vi "Radau5_Step and Stage Value Calculation.vi"(8 "Y(k)":dbl[](array[numeric]), 9 "Increment Z":dbl[](array[numeric]), 10 "Step size":dbl, 11 "Width":i32) -> (0 "Stage value of Y":dbl[][](array[numeric]), 1 "Stage value of Y'":dbl[][](array[numeric]), 2 "Y(k+1) out":dbl[](array[numeric]), 3 "Y'(k+1) out":dbl[](array[numeric]))   [LabVIEW 2020, in "NI_DAE.lvlib"]
uses:
  <vilib>/gmath/NI_DAE.lvlib
  <vilib>/Analysis/Matrix/Datatypes/RealMatrix.ctl
  <vilib>/Analysis/Matrix/Numeric/Multiply/Multiply - RM,R.vi
  <vilib>/Analysis/Matrix/NI_Matrix.lvlib
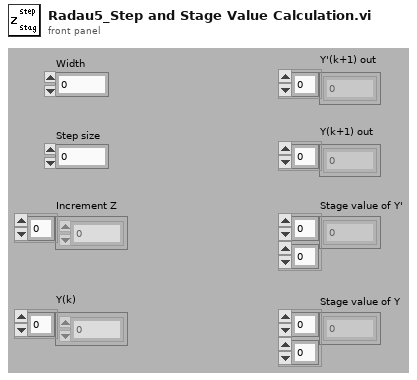
[diagram p1: front panel]
types:
  T1 = typedef "NI_Matrix.lvlib/RealMatrix.ctl" = dbl[][]
  T2 = cluster{"A * c[0]":dbl, "A * c[1]":dbl, "A * c[2]":dbl}
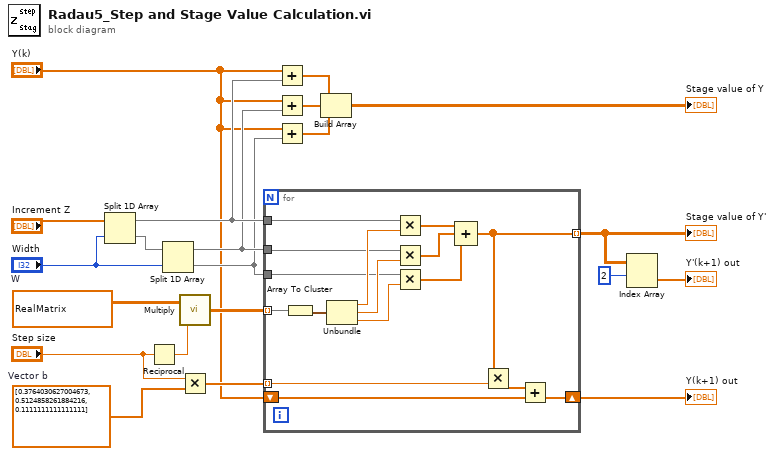
[diagram p0: block diagram]
diagram:
  w8 = dbl[] [0.3764030627004673, 0.5124858261884216, 0.1111111111111111]  # Vector b
  w21 = T1 [[3.2247448713915894, 1.1678400846904053, -0.2531972647421808], [-3.5678400846904057, 0.775255128608411, 1.053197264742181], [5.5319726474218065, -7.53197264742181, 5.0]]  # W
  n1 = Split 1D Array(array="Increment Z", index="Width") -> (first subarray=w15:dbl[], second subarray=w16:dbl[])
  n2 = Reciprocal(x="Step size") -> (1/x=w20:dbl)
  n3 = Split 1D Array(array=w16, index="Width") -> (first subarray=w14:dbl[], second subarray=w13:dbl[])
  n4 = call-poly <vilib>:"Multiply.vi"("Real Scalar c"=w20, "Real Matrix A"=w21) -> ("A * c"=w19:T1)
  n5 = Multiply(x="Step size", y=w8) -> (x*y=w7:dbl[])
  n6 = for {
    tunnel: w19 -> [w37] mode=indexing
    tunnel: w15 -> [w33]
    tunnel: w14 -> [w34]
    tunnel: w13 -> [w31]
    tunnel: [w25] -> w4 mode=indexing
    tunnel: w7 -> [w26] mode=indexing
    shift-right: [w23] -> w5
    shift-left: "Y(k)" -> [w22]
    n7 = Array To Cluster(array=w37) -> (cluster=w36:T2)
    n8 = Unbundle(w36) -> ("A * c[0]"=w35:dbl, "A * c[1]"=w32:dbl, "A * c[2]"=w30:dbl)
    n9 = Multiply(x=w33, y=w35) -> (x*y=w29:dbl[])
    n10 = Multiply(x=w34, y=w32) -> (x*y=w28:dbl[])
    n11 = Multiply(x=w31, y=w30) -> (x*y=w27:dbl[])
    n12 = Compound Arithmetic op=ADD(w29, w28, w27) -> (w25:dbl[])
    n13 = Multiply(x=w25, y=w26) -> (x*y=w24:dbl[])
    n14 = Add(x=w24, y=w22) -> (x+y=w23:dbl[])
  }
  "Stage value of Y'" <- w4
  "Y(k+1) out" <- w5
  n15 = Add(x="Y(k)", y=w15) -> (x+y=w12:dbl[])
  n16 = Add(x="Y(k)", y=w14) -> (x+y=w11:dbl[])
  n17 = Add(x="Y(k)", y=w13) -> (x+y=w10:dbl[])
  n18 = Build Array(w12, w11, w10) -> (→"Stage value of Y":dbl[][])
  n19 = Index Array(array=w4, index (row)=2) -> (element=→"Y'(k+1) out":dbl[])  [unwired: 1 in]
